vi "GetAlarms.vi"(0 "Signal in":refnum<class "Signal.lvclass">, 11 "error in (no error)":errorcluster) -> (4 "Signal out":refnum<class "Signal.lvclass">, 6 "Alarm":bool, 8 "Warning":bool, 15 "error out":errorcluster)   [LabVIEW 2019, in "Signal.lvclass"]
uses:
  Signal.lvclass
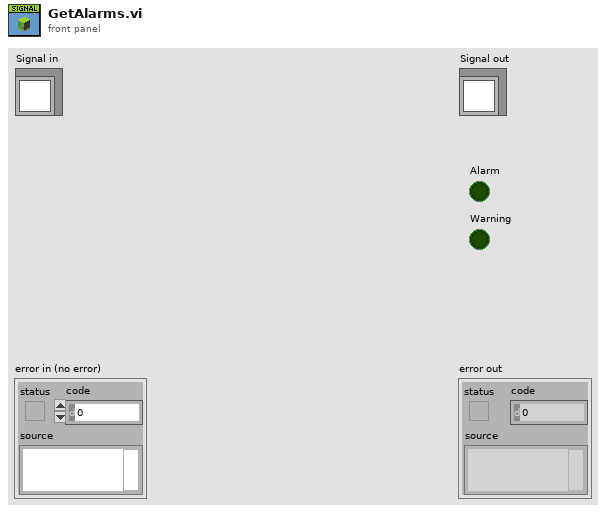
[diagram p1: front panel]
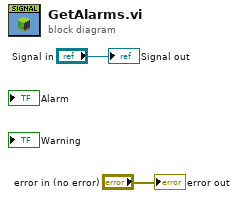
[diagram p0: block diagram]
diagram:
  "error out" <- "error in (no error)"
  "Signal out" <- "Signal in"
